vi "Write.vi"(8 "error in (no error)":errorcluster, 10 "Value":T1, 11 "Boolean in":refnum<class "SynchType_U64.lvclass">) -> (0 "error out":errorcluster, 3 "Boolean out":refnum<class "SynchType_U64.lvclass">)   [LabVIEW 2021, in "BT.lvlib" / "SynchType_U64.lvclass"]
doc: "Abstract Data Classes 2.1.1.12\nTim Streeter - TSA\nCopyright (c) 2024, TSA"
uses:
  SynchType_U64.lvclass
  SynchType_U64.lvclass/SynchType_U64.ctl
  Type.ctl
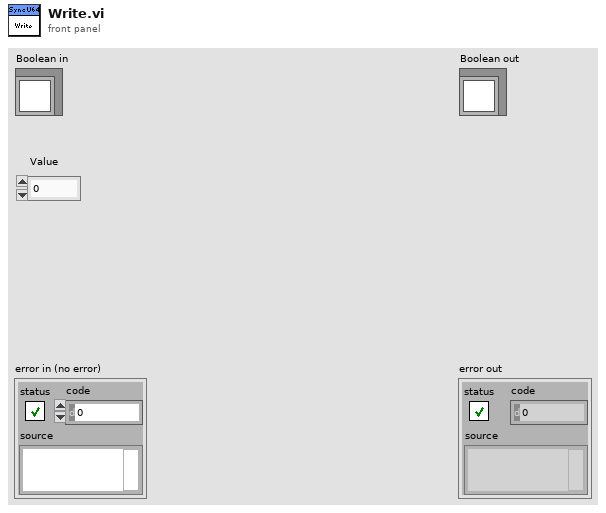
[diagram p1: front panel]
types:
  T1 = typedef "BT.lvlib/SynchType_U64.lvclass/Type.ctl" = u32
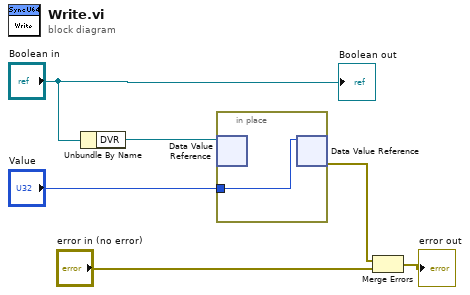
[diagram p0: block diagram]
diagram:
  n1 = Unbundle By Name("Boolean in") -> ("DVR"=w3:refnum<data-value>)
  n2 = in-place {
    in-place-border: "Value" -> [w7]
    n3 = in-place-dvr #1(w3) -> ()  [unwired: 2 out]
    n4 = in-place-dvr #1(w7) -> (w1:errorcluster)  [unwired: 1 out]
  }
  n5 = Merge Errors(w1, "error in (no error)") -> (→"error out":errorcluster)
  "Boolean out" <- "Boolean in"
